vi "runscenario get items from POST.vi"(5 "POST (empty)":T3) -> (1 "Generator Settings":T1={"Wait? (t)"=TRUE, "ClientPrint? (f)"=FALSE, "Client (\"\")"="", "joinPDF"=FALSE, "Sort Method"=enum."Item", "Export Row (-1=all)"=-1, "Preview"=FALSE, "Estimate Time"=FALSE, "username"="", "jobid"=""}, 2 "Items":T2[](array[typedef]))   [LabVIEW 2011]
uses:
  ITK EXT/utils/keyedarr.llb/Keyed Array.ctl
  _cgi-lib/TDM_INDEX Record.ctl
  server/DIAdem/Datasheet/Datasheet Generator Settings.ctl
  ITK EXT/utils/strutil.llb/Case Matching.ctl
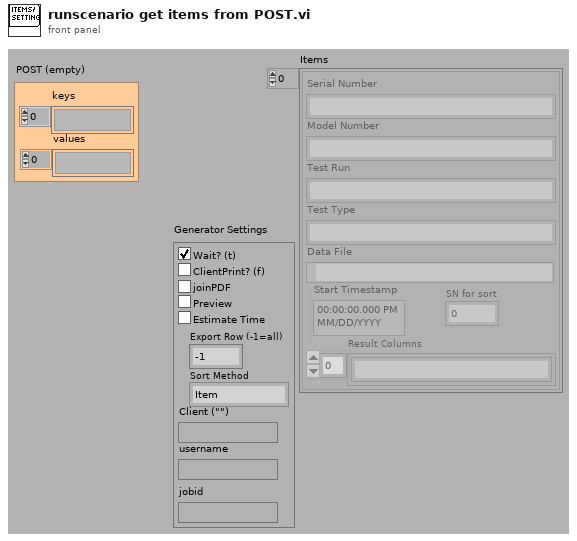
[diagram p1: front panel]
types:
  T1 = typedef "DATASHEET Generator Settings.ctl" = cluster{"Wait? (t)":bool, "ClientPrint? (f)":bool, "Client (\"\")":string, "joinPDF":bool, "Sort Method":enum16{"Item", "Template", "No Sort"}, "Export Row (-1=all)":i32, "Preview":bool, "Estimate Time":bool, "username":string, "jobid":string}
  T2 = typedef "TDM_INDEX Record.ctl" = cluster{"Model Number":string, "SN for sort":i32, "Test Type":string, "Test Run":string, "Serial Number":string, "Start Timestamp":timestamp, "Data File":path, "Result Columns":string[]}
  T3 = typedef "Keyed Array.ctl" = cluster{"keys":string[], "values":string[]}
  T4 = typedef "Case Matching.ctl" = enum16{"a != A", "a == A", "system"}
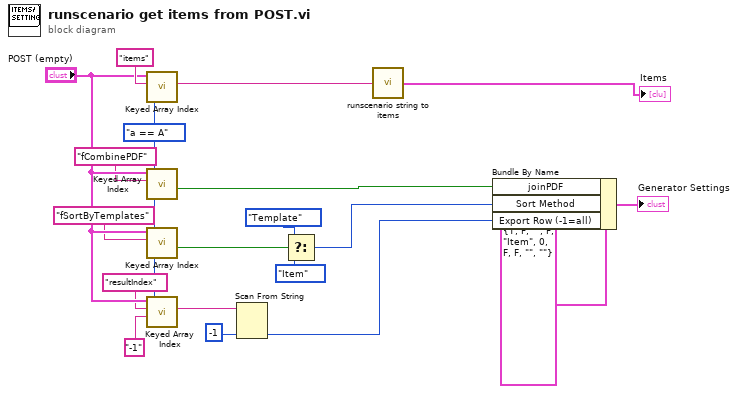
[diagram p0: block diagram]
diagram:
  w13 = Case_Matching."a == A" ("case matching (sensitive)")
  n1 = call "Keyed Array Index.vi"("case matching (sensitive)"=w13, "key"="items" ("Template (\"\")"), "array in"="POST (empty)") -> ("value"=w19:string)  [unwired: 1 in, 3 out]
  n2 = call "Keyed Array Index.vi"("case matching (sensitive)"=w13, "key"="fCombinePDF" ("Template (\"\")"), "array in"="POST (empty)") -> ("valid key"=w11:bool)  [unwired: 1 in, 3 out]
  n3 = call "Keyed Array Index.vi"("case matching (sensitive)"=w13, "key"="fSortByTemplates" ("Template (\"\")"), "array in"="POST (empty)") -> ("valid key"=w1:bool)  [unwired: 1 in, 3 out]
  n4 = call "Keyed Array Index.vi"("case matching (sensitive)"=w13, "default value"="-1", "key"="resultIndex" ("Template (\"\")"), "array in"="POST (empty)") -> ("value"=w7:string)  [unwired: 3 out]
  n5 = Scan From String(input string=w7, default 1=-1 ("Export Row (-1=all)")) -> (output 1=w5:i32)  [unwired: 3 in, 3 out]
  n6 = Select(t=enum16{"Item", "Template", "No Sort"}."Template" ("Sort Method"), s=w1, f=enum16{"Item", "Template", "No Sort"}."Item" ("Sort Method")) -> (s? t:f=w3:enum16{"Item", "Template", "No Sort"})
  n7 = call "runscenario string to items.vi"("value"=w19) -> ("Items"=→"Items":T2[])
  n8 = Bundle By Name(cluster=T1 {"Wait? (t)"=TRUE, "ClientPrint? (f)"=FALSE, "Client (\"\")"="", "joinPDF"=FALSE, "Sort Method"=enum."Item", "Export Row (-1=all)"=0, "Preview"=FALSE, "Estimate Time"=FALSE, "username"="", "jobid"=""} ("Generator Settings"), "joinPDF"=w11, "Sort Method"=w3, "Export Row (-1=all)"=w5) -> (→"Generator Settings":T1)
